vi "Read Snake Status Remote.vi"(8 "error in (no error)":errorcluster, 11 "Snake in":refnum<class "Snake.lvclass">) -> (0 "error out":errorcluster, 3 "Snake Status":T1)   [LabVIEW 2021, in "Snake.lvclass"]
uses:
  Snake.lvclass
  Snake Status.ctl
  Snake.lvclass/Snake.ctl
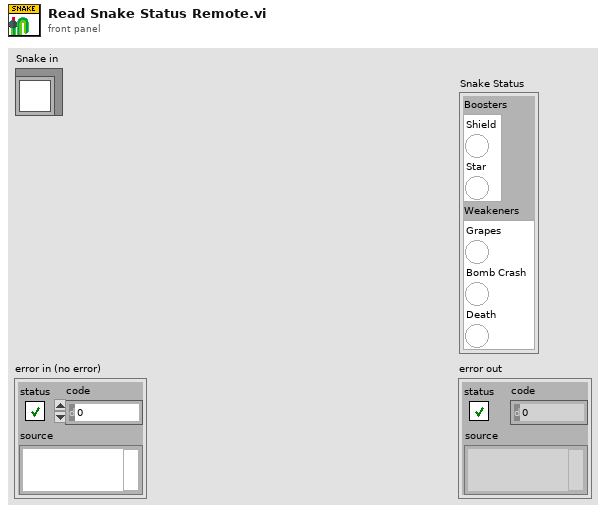
[diagram p1: front panel]
types:
  T1 = typedef "Snake.lvclass/Snake Status.ctl" = cluster{"Boosters":cluster{"Shield":bool, "Star":bool}, "Weakeners":cluster{"Grapes":bool, "Bomb Crash":bool, "Death":bool}}
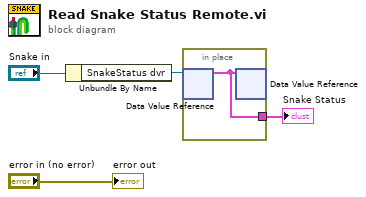
[diagram p0: block diagram]
diagram:
  n1 = Unbundle By Name("Snake in") -> ("SnakeStatus dvr"=w2:refnum<data-value>)
  n2 = in-place {
    in-place-border: [w5] -> w1
    n3 = in-place-dvr #1(w2) -> (w5:T1)  [unwired: 1 out]
    n4 = in-place-dvr #1(w5) -> ()  [unwired: 2 out]
  }
  "Snake Status" <- w1
  "error out" <- "error in (no error)"
